vi "WSVCAP SHL Host LL I2C Convert Hex Reg Values to Capacitance.vi"(0 "Bytes (H-M-L)":u8[](array[numeric]) format="%.0x") -> (4 "Capacitance (pF)":dbl format="%.3f pF")   [LabVIEW 2012]
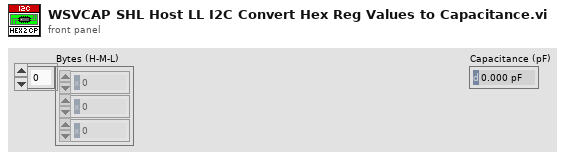
[diagram p1: front panel]
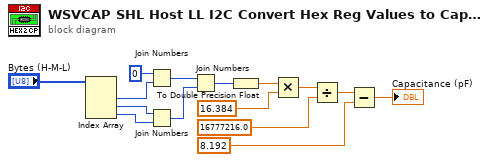
[diagram p0: block diagram]
diagram:
  n1 = Index Array(array="Bytes (H-M-L)") -> (element #1=w14:u8, element #2=w12:u8, element #3=w11:u8)  [unwired: 3 in]
  n2 = Join Numbers(hi=u8 0, lo=w14) -> ((hi.lo)=w10:u16)
  n3 = Join Numbers(hi=w12, lo=w11) -> ((hi.lo)=w9:u16)
  n4 = Join Numbers(hi=w10, lo=w9) -> ((hi.lo)=w8:u32)
  n5 = To Double Precision Float(number=w8) -> (double precision float=w7:dbl)
  n6 = Multiply(x=w7, y=16.384) -> (x*y=w5:dbl)
  n7 = Divide(x=w5, y=16777216.0) -> (x/y=w3:dbl)
  n8 = Subtract(x=w3, y=8.192) -> (x-y=→"Capacitance (pF)":dbl)
